vi "自搭_姿态显示_故障注入.vi"() -> ()   [LabVIEW 2016]
uses:
  <vilib>/Instr/_visa.llb/VISA Configure Serial Port (Instr).vi
panel:
  in  "复位":bool
  in  "暂停":bool
  in  "小数":string
  in  "卡滞发生时间":string
  in  "角度（小数）":string
  in  "卡滞角度":string
  in  "退化故障":string(combo)
  in  "控制方法":string(combo)
  out "X":dbl(graph)
  out "当前时间-秒":dbl
  out "Y":dbl(graph)
  in  "波特率":dbl
  in  "故障腿":string(combo)
  in  "data bits (8)":u16=8 caption="数据比特(8)" min=5 max=8 step=1
  in  "arduino端口":refnum<visa-resource-name>
  in  "控制程序启动":bool
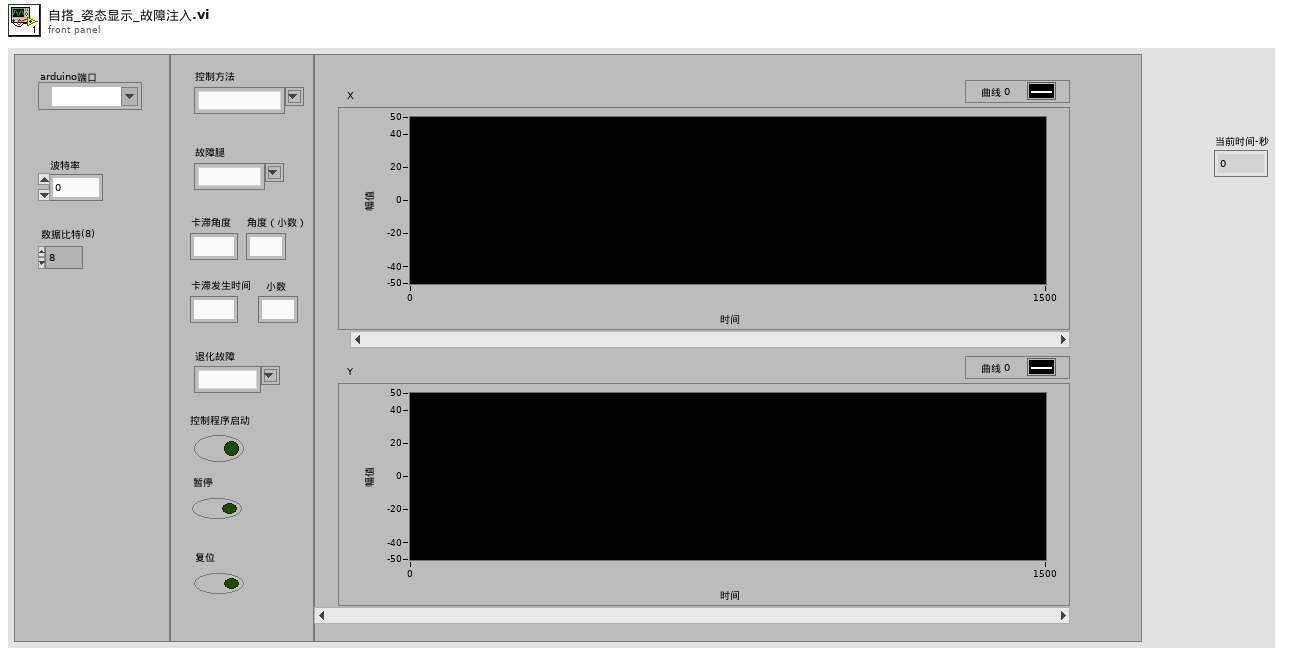
[diagram p1: front panel]
types:
  T1 = typedef "LVDateTimeRec.ctl" = cluster{"秒数的小数部分":dbl, "秒":i32, "分":i32, "时":i32, "日":i32, "月":i32, "年":i32, "天数（周）":i32, "天数（年）":i32, "DST":i32}
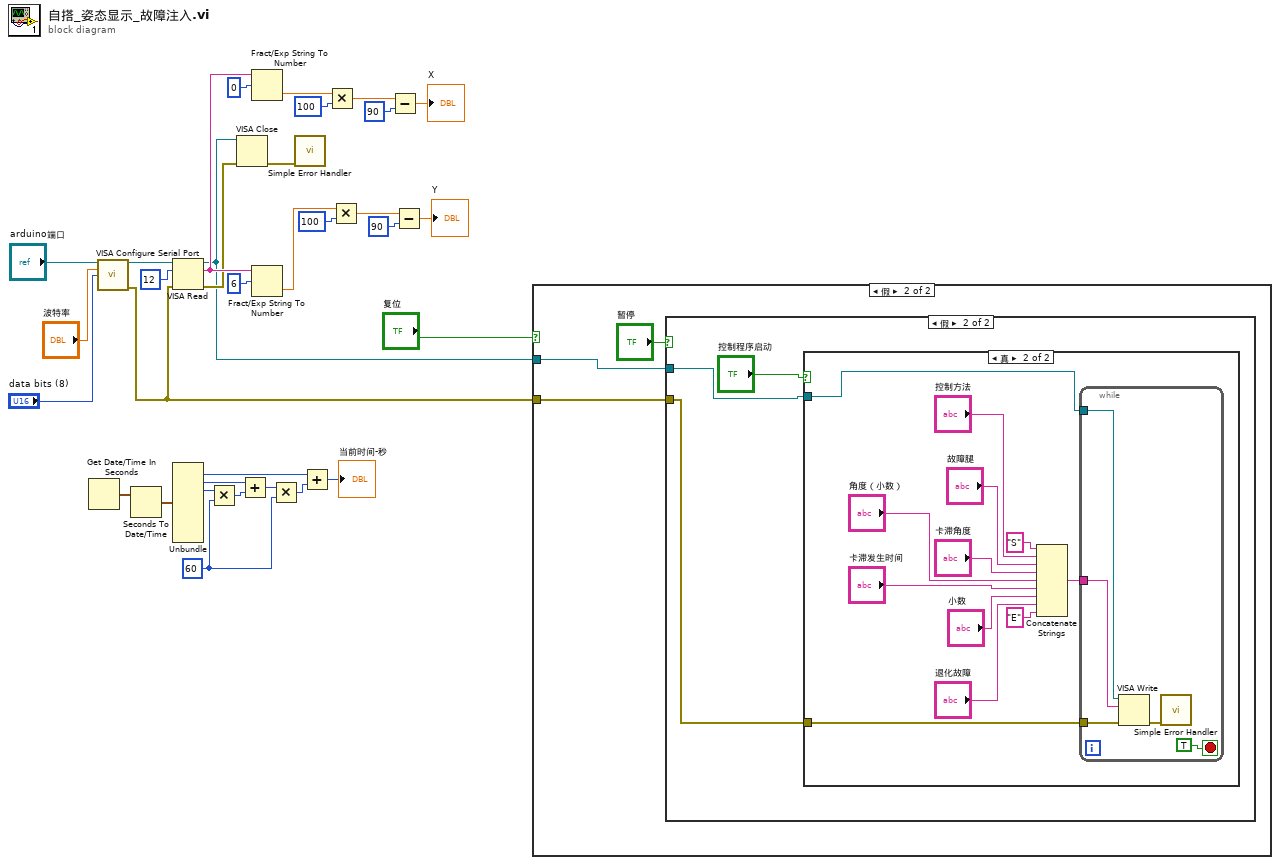
[diagram p0: block diagram]
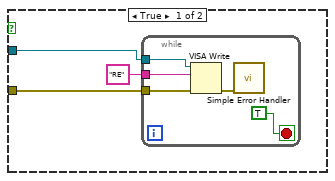
[diagram p2: hidden frame]
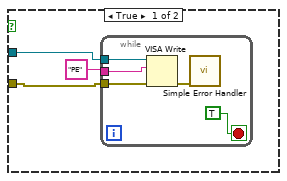
[diagram p3: hidden frame]
diagram:
  w9 = 60
  n1 = Get Date/Time In Seconds() -> (seconds since 1Jan1904=w15:timestamp)
  n2 = call-poly "VISA Configure Serial Port"("VISA resource name"="arduino端口", "baud rate (9600)"="波特率", "data bits (8)"="data bits (8)") -> ("VISA resource name out"=w30:refnum<visa-resource-name>, "error out"=w2:errorcluster)  [unwired: 11 in]
  n3 = Seconds To Date/Time(time stamp (now)=w15) -> (date time rec=w14:T1)  [unwired: 1 in]
  n4 = VISA Read(VISA resource name=w30, byte count=12, error in (no error)=w2) -> (VISA resource name out=w3:refnum<visa-resource-name>, read buffer=w18:string, error out=w16:errorcluster)  [unwired: 1 out]
  n5 = Unbundle(w14) -> ("秒"=w7:i32, "分"=w11:i32, "时"=w13:i32)  [unwired: 7 out]
  n6 = Multiply(x=w13, y=w9) -> (x*y=w12:i32)
  n7 = VISA Close(VISA resource name=w3, error in (no error)=w16) -> (error out=w17:errorcluster)
  n8 = Add(x=w11, y=w12) -> (x+y=w10:i32)
  n9 = Fract/Exp String To Number(string=w18, offset=0) -> (number=w27:dbl)  [unwired: 3 out]
  n10 = Fract/Exp String To Number(string=w18, offset=6) -> (number=w22:dbl)  [unwired: 3 out]
  n11 = Multiply(x=w10, y=w9) -> (x*y=w6:i32)
  n12 = call <vilib>:"Simple Error Handler.vi"("error in (no error)"=w17) -> ()  [unwired: 1 in, 8 out]
  n13 = Add(x=w7, y=w6) -> (x+y=→"当前时间-秒":i32)
  n14 = Multiply(x=w27, y=100) -> (x*y=w25:dbl)
  n15 = Multiply(x=w22, y=100) -> (x*y=w20:dbl)
  n16 = Subtract(x=w25, y=90) -> (x-y=→"X":dbl)
  n17 = Subtract(x=w20, y=90) -> (x-y=→"Y":dbl)
  n18 = case shown="假" "复位" {
    tunnel: w3 -> [w36 w44]
    tunnel: w2 -> [w35 w43]
    frame True {
      n19 = while {
        tunnel: w36 -> [w39]
        tunnel: "RE" -> [w38]
        tunnel: w35 -> [w37]
        stop <- TRUE stop-if-true
        n20 = VISA Write(VISA resource name=w39, write buffer=w38, error in (no error)=w37) -> (error out=w40:errorcluster)  [unwired: 2 out]
        n21 = call <vilib>:"Simple Error Handler.vi"("error in (no error)"=w40) -> ()  [unwired: 1 in, 8 out]
      }
    }
    frame False {
      n22 = case shown="假" "暂停" {
        tunnel: w44 -> [w47 w55]
        tunnel: w43 -> [w46 w53]
        frame True {
          n23 = while {
            tunnel: w47 -> [w50]
            tunnel: "PE" -> [w49]
            tunnel: w46 -> [w48]
            stop <- TRUE stop-if-true
            n24 = VISA Write(VISA resource name=w50, write buffer=w49, error in (no error)=w48) -> (error out=w51:errorcluster)  [unwired: 2 out]
            n25 = call <vilib>:"Simple Error Handler.vi"("error in (no error)"=w51) -> ()  [unwired: 1 in, 8 out]
          }
        }
        frame False {
          n26 = case shown="真" "控制程序启动" {
            tunnel: w55 -> [_ w58]
            tunnel: w53 -> [_ w56]
            frame False {
            }
            frame True {
              n27 = Concatenate Strings("S", "控制方法", "故障腿", "卡滞角度", "角度（小数）", "卡滞发生时间", "小数", "退化故障", "E") -> (w57:string)
              n28 = while {
                tunnel: w58 -> [w70]
                tunnel: w57 -> [w69]
                tunnel: w56 -> [w68]
                stop <- TRUE stop-if-true
                n29 = VISA Write(VISA resource name=w70, write buffer=w69, error in (no error)=w68) -> (error out=w71:errorcluster)  [unwired: 2 out]
                n30 = call <vilib>:"Simple Error Handler.vi"("error in (no error)"=w71) -> ()  [unwired: 1 in, 8 out]
              }
            }
          }
        }
      }
    }
  }
